vi "FindBlob_ReNum.vi"(1 "duplicates":T1(array[cluster]), 2 "Image Data in":u32[](array[numeric])) -> (0 "Image Data out":u32[](array[numeric]))   [LabVIEW 2024]
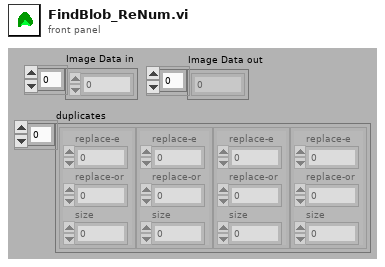
[diagram p1: front panel]
types:
  T1 = cluster{"replace-e":u32, "replace-or":u32, "size":u32}[]
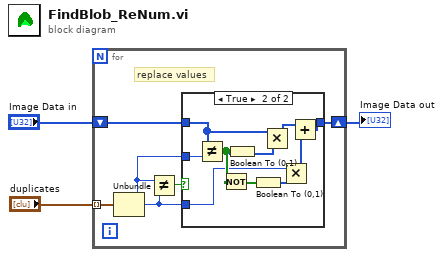
[diagram p0: block diagram]
diagram:
  n1 = for {
    shift-right: [w7] -> w1
    shift-left: "Image Data in" -> [w8]
    tunnel: "duplicates" -> [w9] mode=indexing
    # "replace values"
    n2 = Unbundle(w9) -> ("replace-e"=w6:u32, "replace-or"=w4:u32)  [unwired: 1 out]
    n3 = Not Equal?(x=w6, y=w4) -> (x != y?=w5:bool)
    n4 = case shown="True" w5 {
      tunnel: w8 -> [w10 w20]
      tunnel: [w10 w15] -> w7
      tunnel: w6 -> [_ w12]
      tunnel: w4 -> [_ w11]
      frame False {
      }
      frame True {
        n5 = Not Equal?(x=w20, y=w12) -> (x != y?=w14:bool[])
        n6 = Not(x=w14) -> (.not. x?=w18:bool[])
        n7 = Boolean To (0,1)(Boolean=w14) -> (0, 1=w19:i16[])
        n8 = Boolean To (0,1)(Boolean=w18) -> (0, 1=w13:i16[])
        n9 = Multiply(x=w20, y=w19) -> (x*y=w17:u32[])
        n10 = Multiply(x=w11, y=w13) -> (x*y=w16:u32[])
        n11 = Add(x=w17, y=w16) -> (x+y=w15:u32[])
      }
    }
  }
  "Image Data out" <- w1
